vi "Serial_Lvl_Read.vi"(8 "error in (no error)":errorcluster, 11 "VISA Refnum in":refnum<visa-resource-name>) -> (0 "error out":errorcluster, 1 "Numeric":u32, 2 "read buffer":string, 3 "VISA Refnum out":refnum<visa-resource-name>)   [LabVIEW 2020, in "GPP.lvlib"]
uses:
  GPP.lvlib
panel:
  out "Array":u32[](array[numeric])
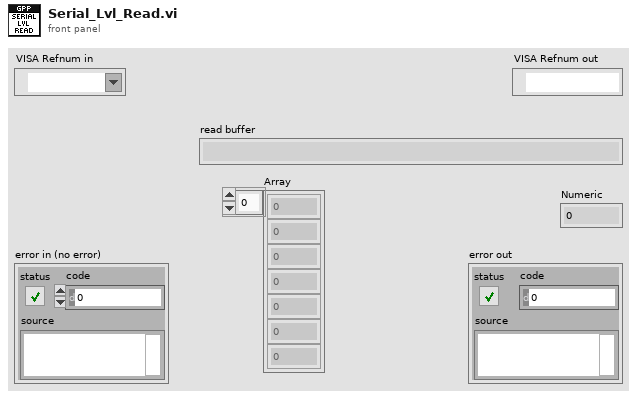
[diagram p1: front panel]
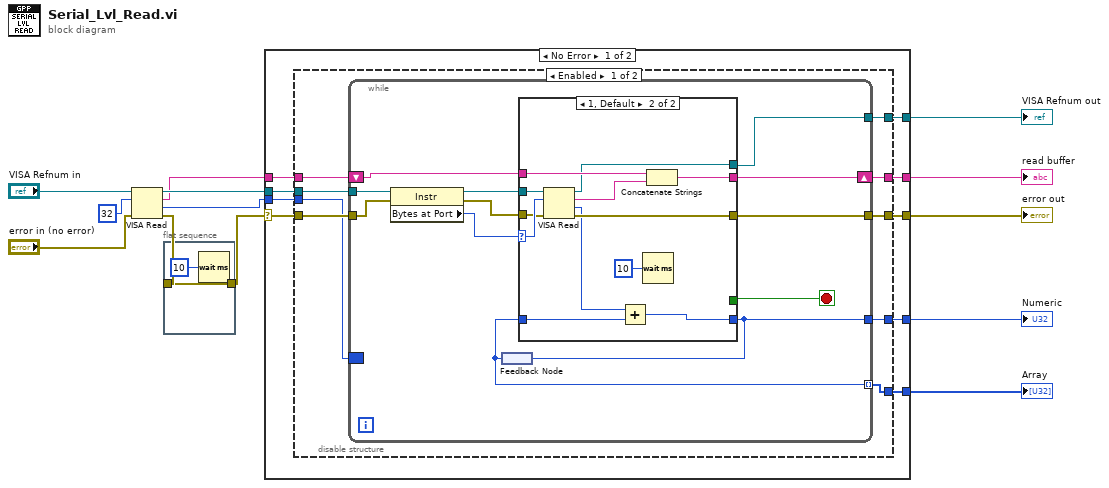
[diagram p0: block diagram]
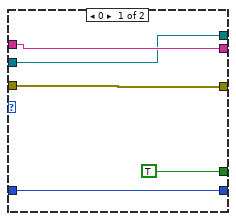
[diagram p2: hidden frame]
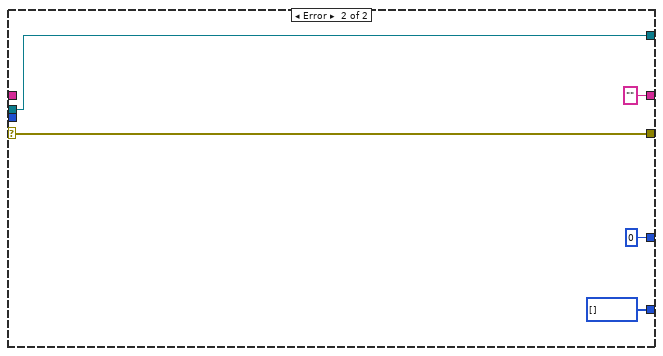
[diagram p4: hidden frame]
diagram:
  n1 = VISA Read(VISA resource name="VISA Refnum in", byte count=u32 32, error in (no error)="error in (no error)") -> (VISA resource name out=w9:refnum<visa-resource-name>, read buffer=w7:string, return count=w8:u32, error out=w4:errorcluster)
  n2 = flat-sequence {
    tunnel: [w15] -> w3
    tunnel: w4 -> [w15]
    frame #0 {
      n3 = Wait (ms)(milliseconds to wait=u32 10) -> ()  [unwired: 1 out]
    }
  }
  n4 = case shown="No Error" w3 {
    selector: w3 -> [w16 w66]
    tunnel: [w24 w66] -> w1
    tunnel: [w23 u32 0] -> w13
    tunnel: [w22 "" ("read buffer")] -> w12
    tunnel: [w21 w67] -> w11
    tunnel: w9 -> [w20 w67]
    tunnel: w8 -> [w19 _]
    tunnel: w7 -> [w18 _]
    tunnel: [w17 u32[] []] -> w5
    frame No Error {
      n5 = disable-structure shown="Enabled" {
        disable-tunnel: [w33 w63] -> w24
        disable-tunnel: [w32 _] -> w23
        disable-tunnel: [w31 w65] -> w22
        disable-tunnel: [w30 w64] -> w21
        disable-tunnel: w20 -> [w29 w64]
        disable-tunnel: w19 -> [w25 _]
        disable-tunnel: w18 -> [w28 w65]
        disable-tunnel: [w27 _] -> w17
        disable-tunnel: w16 -> [w26 w63]
        frame Enabled {
          n6 = while {
            tunnel: w29 -> [w45]
            border: w25 -> [_]
            tunnel: [w42] -> w32
            shift-right: [w44] -> w31
            shift-left: w28 -> [w43]
            tunnel: [w40] -> w30
            tunnel: [w41] -> w27 mode=indexing
            tunnel: w26 -> [w37]
            tunnel: [w39] -> w33
            stop <- w36 stop-if-true
            n7 = property class="Instr"(reference=w45, error in=w37) -> (reference out=w38:refnum<visa-resource-name>, error out=w34:errorcluster, "Bytes at Port"=w35:u32)
            n8 = feedback #1() -> (w41:u32)
            n9 = case shown="1, Default" w35 {
              selector: w35 -> [_ w53]
              tunnel: w38 -> [w48 w62]
              tunnel: [w46 w55] -> w39
              tunnel: [w50 w61] -> w42
              tunnel: w41 -> [w50 w60]
              tunnel: [w49 w58] -> w44
              tunnel: w43 -> [w49 w57]
              tunnel: [w48 w56] -> w40
              tunnel: [TRUE _] -> w36
              tunnel: w34 -> [w46 w52]
              frame 0 {
              }
              frame 1, Default {
                n10 = VISA Read(VISA resource name=w62, byte count=w53, error in (no error)=w52) -> (VISA resource name out=w56:refnum<visa-resource-name>, read buffer=w59:string, return count=w54:u32, error out=w55:errorcluster)
                n11 = Add(x=w54, y=w60) -> (x+y=w61:u32)
                n12 = Wait (ms)(milliseconds to wait=u32 10) -> ()  [unwired: 1 out]
                n13 = Concatenate Strings(w57, w59) -> (w58:string)
              }
            }
            n14 = feedback-in #1(w42) -> ()
          }
        }
        frame Disabled {
        }
      }
    }
    frame Error {
    }
  }
  "Numeric" <- w13
  "error out" <- w1
  "read buffer" <- w12
  "VISA Refnum out" <- w11
  "Array" <- w5
